vi "Parse Lon.vi"(9 "E/W Index":i32, 10 "Longitude Index":i32, 11 "Fields In":string[](array[string])) -> (2 "Longitude":dbl format="%#_12f", 3 "Fields":string[](array[string]))   [LabVIEW 2020, in "nmea.lvlib" / "nmea.lvclass"]
uses:
  nmea.lvclass
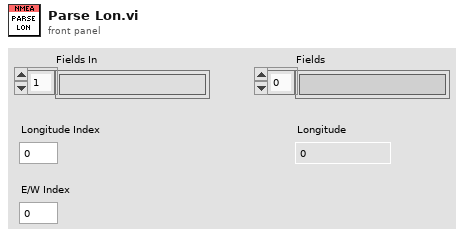
[diagram p1: front panel]
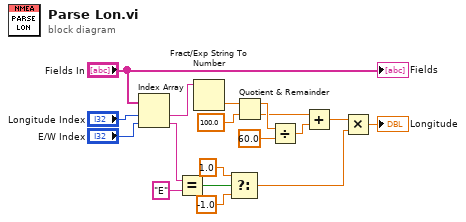
[diagram p0: block diagram]
diagram:
  n1 = Index Array(array="Fields In", index #1="Longitude Index", index #2="E/W Index") -> (element #1=w16:string, element #2=w8:string)
  n2 = Equal?(x=w8, y="E") -> (x = y?=w6:bool)
  n3 = Fract/Exp String To Number(string=w16) -> (number=w14:dbl)  [unwired: 3 in, 1 out]
  n4 = Select(t=1.0, s=w6, f=-1.0 ("t")) -> (s? t:f=w2:dbl)
  n5 = Quotient & Remainder(x=w14, y=100.0) -> (x-y*floor(x/y)=w12:dbl, floor(x/y)=w10:dbl)
  n6 = Divide(x=w12, y=60.0) -> (x/y=w9:dbl)
  n7 = Add(x=w10, y=w9) -> (x+y=w3:dbl)
  n8 = Multiply(x=w3, y=w2) -> (x*y=→"Longitude":dbl)
  "Fields" <- "Fields In"
